vi "addtest.vi"(4 "a":dbl, 6 "b":dbl) -> (7 "c":dbl)   [LabVIEW 2018]
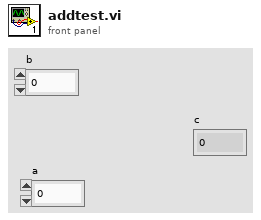
[diagram p1: front panel]
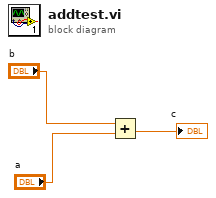
[diagram p0: block diagram]
diagram:
  n1 = Add(x="b", y="a") -> (x+y=→"c":dbl)
